vi "Turn all channels on (SubVI).vi"() -> (3 "String":string)   [LabVIEW 2018]
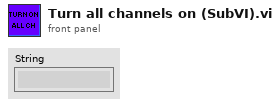
[diagram p1: front panel]
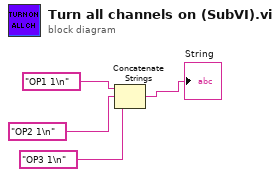
[diagram p0: block diagram]
diagram:
  n1 = Concatenate Strings("OP1 1\n", "OP2 1\n", "OP3 1\n") -> (→"String":string)
